vi "Subvi probe 3 bits DIO29-31 D0-2.vi"(9 "U8":u8) -> ()   [LabVIEW 2017]
uses:
  <vilib>/rvi/eio/common/nirviEmuTemplateMethod_errors.vi
  <vilib>/eio/EIONode/EIONode.xnode
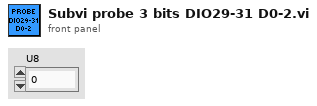
[diagram p1: front panel]
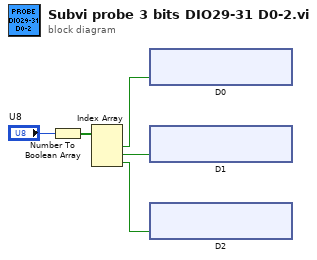
[diagram p0: block diagram]
diagram:
  n1 = Number To Boolean Array(number="U8") -> (Boolean array=w3:bool[])
  n2 = Index Array(array=w3) -> (element #1=w2:bool, element #2=w1:bool, element #3=w4:bool)  [unwired: 3 in]
  n3 = xnode "D0"("Connector0/DIO31"=w2) -> ()  [unwired: 1 in, 1 out]
  n4 = xnode "D1"("Connector0/DIO30"=w1) -> ()  [unwired: 1 in, 1 out]
  n5 = xnode "D2"("Connector0/DIO29"=w4) -> ()  [unwired: 1 in, 1 out]
